vi "global_stop.vi"() -> ()   [LabVIEW 2013]
doc: "A collection of global boolean flags."
panel:
  in  "Poll devices":bool
  in  "Stop":bool
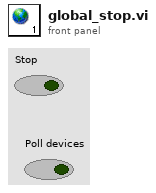
[diagram p1: front panel]
diagram:
